vi "TramepourGBCMOD.vi"(9 "Out":T1, 10 "TestNum":string="TestNub", 11 "SN":string) -> (3 "String":string)   [LabVIEW 2020]
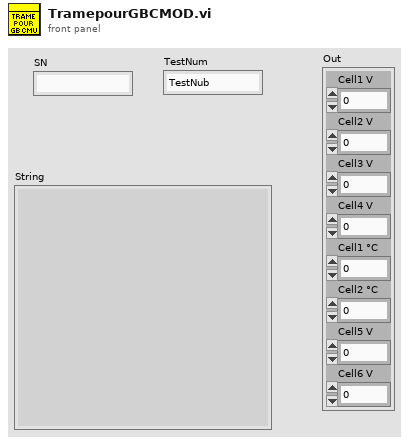
[diagram p1: front panel]
types:
  T1 = cluster{"Cell1 V":sgl, "Cell2 V":sgl, "Cell3 V":sgl, "Cell4 V":sgl, "Cell1 °C":sgl, "Cell2 °C":sgl, "Cell5 V":sgl, "Cell6 V":sgl}
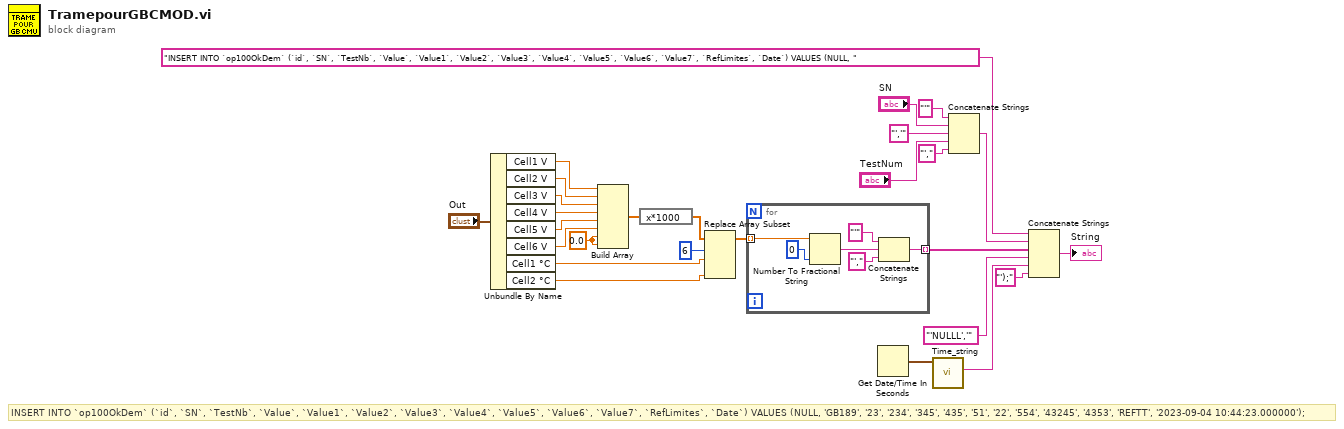
[diagram p0: block diagram]
diagram:
  w25 = sgl 0.0 ("élément")
  # "INSERT INTO `op100OkDem` (`id`, `SN`, `TestNb`, `Value`, `Value1`, `Value2`, `Value3`, `Value4`, `Value5`, `Value6`, `Value7`, `RefLimites`, `Date`) VALUES (NULL, 'GB189', '23', '234', '345', '435', '51', '22', '554', '43245', '4353', 'REFTT', '2023-09-04 10:44:23.000000');"
  n1 = Unbundle By Name("Out") -> ("Cell1 V"=w23:sgl, "Cell2 V"=w22:sgl, "Cell3 V"=w21:sgl, "Cell4 V"=w20:sgl, "Cell5 V"=w19:sgl, "Cell6 V"=w18:sgl, "Cell1 °C"=w14:sgl, "Cell2 °C"=w1:sgl)
  n2 = Build Array(w23, w22, w21, w20, w19, w18, w25, w25) -> (w17:sgl[])
  n3 = expression code="x*1000"(w17) -> (w16:sgl[])
  n4 = Replace Array Subset(array=w16, new element #1=w14, index #1=6 ("indice"), new element #2=w1) -> (w13:sgl[])  [unwired: 1 in]
  n5 = for {
    tunnel: w13 -> [w33] mode=indexing
    tunnel: [w30] -> w9 mode=indexing
    n6 = Number To Fractional String ("Nombre en chaîne fractionnaire")(number=w33, precision (6)=i16 0 ("précision (6)")) -> (F-format string=w29:string)  [unwired: 2 in]
    n7 = Concatenate Strings("'" ("chaîne"), w29, "'," ("string")) -> (w30:string)
  }
  n8 = Get Date/Time In Seconds() -> (seconds since 1Jan1904=w10:timestamp)
  n9 = call <userlib>:"Time_string.vi"("h in"=w10) -> ("heure sql"=w7:string)  [unwired: 9 in, 1 out]
  n10 = Concatenate Strings("'" ("string"), "SN", "','" ("string"), "TestNum", "'," ("string")) -> (w12:string)
  n11 = Concatenate Strings("INSERT INTO `op100OkDem` (`id`, `SN`, `TestNb`, `Value`, `Value1`, `Value2`, `Value3`, `Value4`, `Value5`, `Value6`, `Value7`, `RefLimites`, `Date`) VALUES (NULL, " ("chaîne"), w12, w9, "'NULLL','" ("string"), w7, "');" ("string")) -> (→"String":string)
